vi "No Trip Tests at 120mA old.vi"(3 "error in":errorcluster) -> (10 "error out":errorcluster)   [LabVIEW 2015]
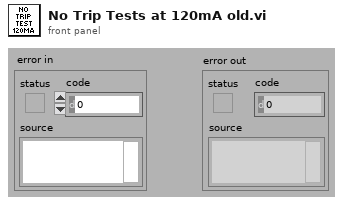
[diagram p1: front panel]
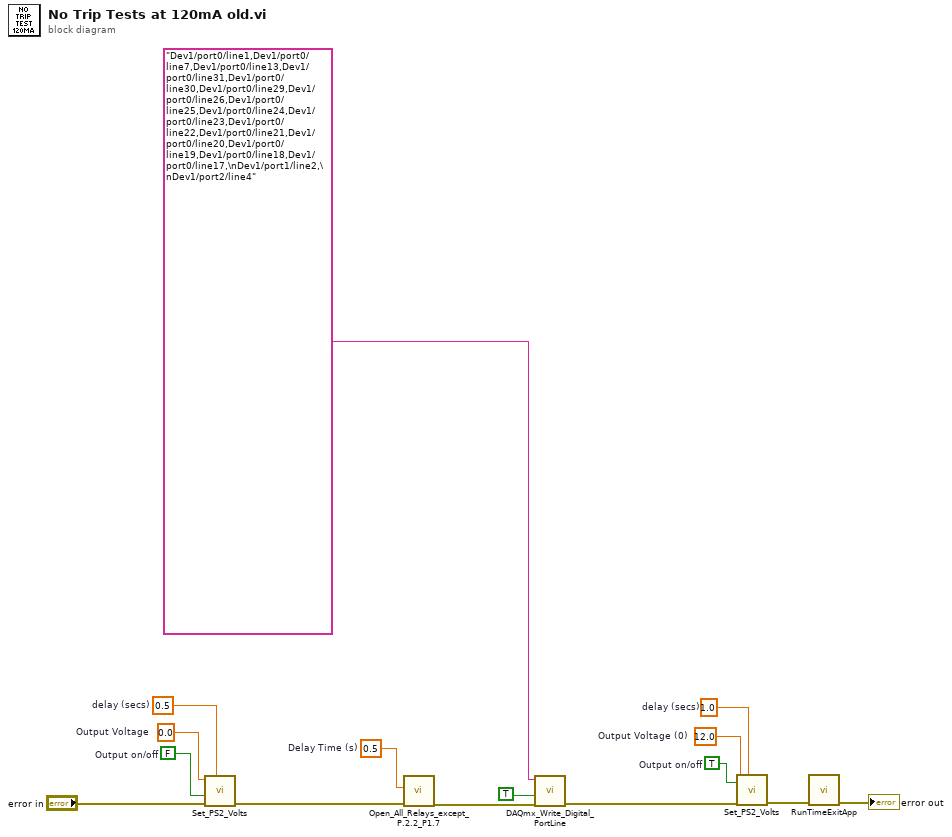
[diagram p0: block diagram]
diagram:
  w1 = 0.5  # Delay Time (s)
  w2 = 0.0  # Output Voltage
  w3 = 0.5  # delay (secs)
  w4 = FALSE  # Output on/off
  w6 = TRUE  # Output on/off
  w9 = 1.0  # delay (secs)
  w11 = 12.0  # Output Voltage (0)
  n1 = call "Set_PS2_Volts.vi"("delay (secs)"=w3, "error in"="error in", "Output on/off"=w4, "Output Voltage"=w2) -> ("error out"=w5:errorcluster)  [unwired: 5 in, 2 out]
  n2 = call "Open_All_Relays_except_P.2.2_P1.7.vi"("Delay Time (s)"=w1, "error in"=w5) -> ("error out"=w7:errorcluster)  [unwired: 7 in]
  n3 = call "DAQmx_Write_Digital_PortLine.vi"("Device/Ports/Lines"="Dev1/port0/line1,Dev1/port0/line7,Dev1/port0/line13,Dev1/port0/line31,Dev1/port0/line30,Dev1/port0/line29,Dev1/port0/line26,Dev1/port0/line25,Dev1/port0/line24,Dev1/port0/line23,Dev1/port0/line22,Dev1/port0/line21,Dev1/port0/line20,Dev1/port0/line19,Dev1/port0/line18,Dev1/port0/line17,\nDev1/port1/line2,\nDev1/port2/line4", "Boolean"=TRUE, "error in"=w7) -> ("error out"=w13:errorcluster)  [unwired: 6 in, 1 out]
  n4 = call "Set_PS2_Volts.vi"("delay (secs)"=w9, "error in"=w13, "Output on/off"=w6, "Output Voltage"=w11) -> ("error out"=w12:errorcluster)  [unwired: 5 in, 2 out]
  n5 = call "RunTimeExitApp.vi"("error in (no error)"=w12) -> ("error out"=→"error out":errorcluster)  [unwired: 10 in]
